vi "Get Model.vi"(8 "error in (no error)":errorcluster, 11 "Simulated Waveform in":refnum<class "Simulated Waveform.lvclass">) -> (0 "error out":errorcluster, 2 "Model":string, 3 "Simulated Waveform out":refnum<class "Simulated Waveform.lvclass">)   [LabVIEW 2020, in "Simulated Waveform.lvlib" / "Simulated Waveform.lvclass"]
uses:
  Simulated Waveform.lvclass
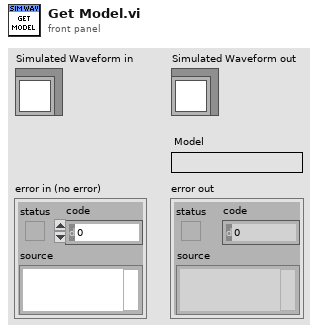
[diagram p1: front panel]
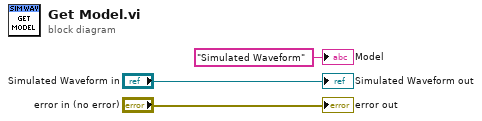
[diagram p0: block diagram]
diagram:
  "error out" <- "error in (no error)"
  "Simulated Waveform out" <- "Simulated Waveform in"
  "Model" <- "Simulated Waveform" ("Model")
